vi "Strip filename base and extension.vi"(0 "Path":path=path "C:/myfiles.are.here.Text") -> (1 "stripped path":path, 2 "Filename base":string="myfiles.are.here", 3 "Filename extension (.txt)":string=".Text")   [LabVIEW 2010]
doc: "This .vi strips the extension from the input file."
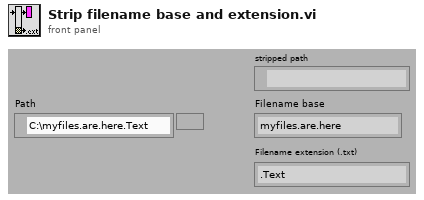
[diagram p1: front panel]
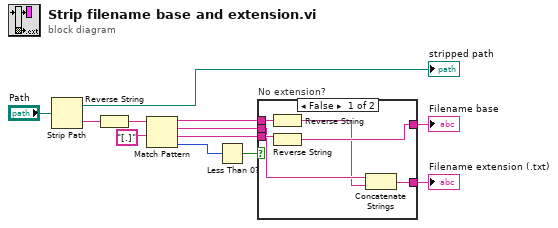
[diagram p0: block diagram]
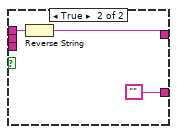
[diagram p2: hidden frame]
diagram:
  n1 = Strip Path(path="Path") -> (stripped path=→"stripped path":path, name=w11:string)
  n2 = Reverse String(1:w11) -> (0:w10:string)
  n3 = Match Pattern(string=w10, regular expression="[.]") -> (before substring=w8:string, match substring=w4:string, after substring=w7:string, offset past match=w2:i32)  [unwired: 1 out]
  n4 = Less Than 0?(x=w2) -> (x < 0?=w1:bool)
  n5 = case "No extension?" shown="False" w1 {
    tunnel: w8 -> [w18 w20]
    tunnel: w7 -> [w17 _]
    tunnel: [w16 w19] -> w6
    tunnel: [w15 ""] -> w5
    tunnel: w4 -> [w14 _]
    frame False {
      n6 = Reverse String(1:w18) -> (0:w13:string)
      n7 = Reverse String(1:w17) -> (0:w16:string)
      n8 = Concatenate Strings(w14, w13) -> (w15:string)
    }
    frame True {
      n9 = Reverse String(1:w20) -> (0:w19:string)
    }
  }
  "Filename base" <- w6
  "Filename extension (.txt)" <- w5
